vi "Circus PCs IPs.vi"(3 "error in (no error)":errorcluster, 4 "ID":string) -> (0 "error out":errorcluster, 1 "IP":string)   [LabVIEW 2026, in "TALOS.lvlib"]
doc: "This VI gives the IP of a PC, given its name, if it has been correctly inserted in the AEgIS_Config_Param.ini. If not present, it returns its ID (which is also its DNS name)."
uses:
  TALOS.lvlib
  Ancestor/Ancestor/Ancestor.lvclass/Ancestor.ctl
  Circus Root Path.vi
  TALOS Config Param.vi
  FGV/Error Memory/Get Error Description.vi
  Get PC name.vi
  Ancestor/Ancestor/Read ID.vi
  Get Class Name.vi
  <vilib>/Utility/error.llb/Clear Errors.vi
  FGV/Error Memory/Error Memory Core.vi
  <vilib>/AdvancedString/Delimited String to 1D String Array.vi
  <vilib>/AdvancedString/Delimited String to 1D String Array (string).vi
  FGV/Error Memory/Error Crt Lvl checker.vi
  FGV/Error Memory/Error Memory Core.vi/40c8088d-b597-4017-91af-faa98e00292e.vi
  FGV/Error Memory/Error Memory Core.vi/d4a3ab98-063c-4e44-b43d-fbdcfe6c2be2.vi
  Global Memory.vi
  <vilib>/Utility/LVClass/Get LV Class Name.vi
  Is in Packed Library.vi
  TALOS Root path.vi
  Read CSV worksheet.vi
  Global Constants.vi
  <vilib>/Utility/error.llb/General Error Handler.vi
  <vilib>/Utility/config.llb/Open Config Data.vi
  <vilib>/Utility/config.llb/Get Section Names.vi
  <vilib>/Utility/config.llb/Get Key Names.vi
  <vilib>/Utility/config.llb/Read Key.vi
  <vilib>/Utility/config.llb/Read Key (String).vi
  <vilib>/Utility/config.llb/Close Config Data.vi
  Ancestor/Ancestor/Ancestor.lvclass
  <vilib>/Comparison/Equal/Equal Functor/Equal Functor.lvclass
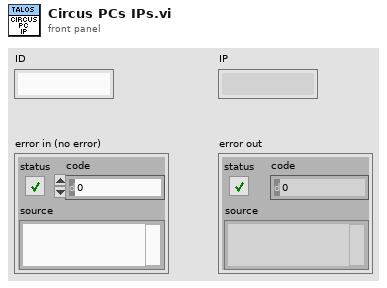
[diagram p1: front panel]
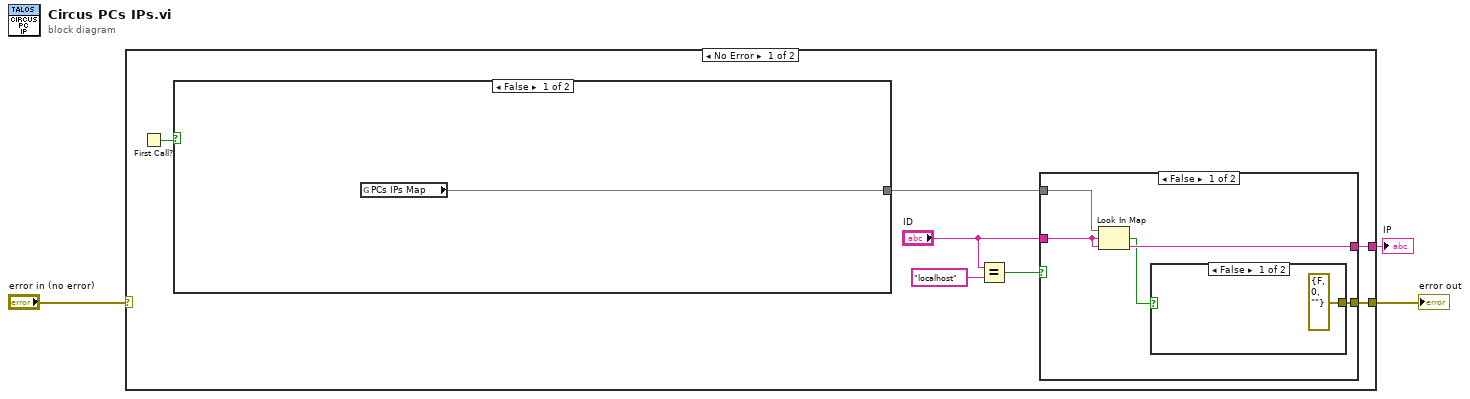
[diagram p0: block diagram]
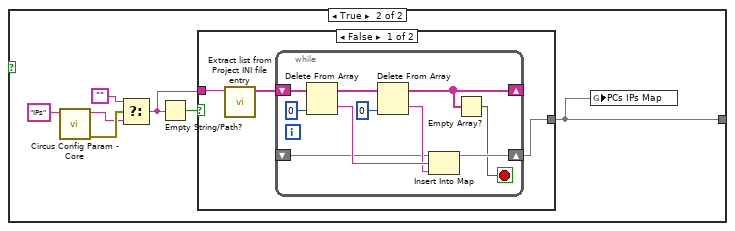
[diagram p2: hidden frame]
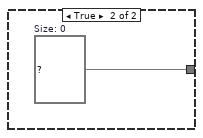
[diagram p3: hidden frame]
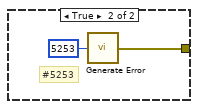
[diagram p4: hidden frame]
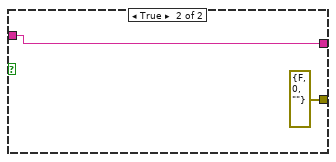
[diagram p5: hidden frame]
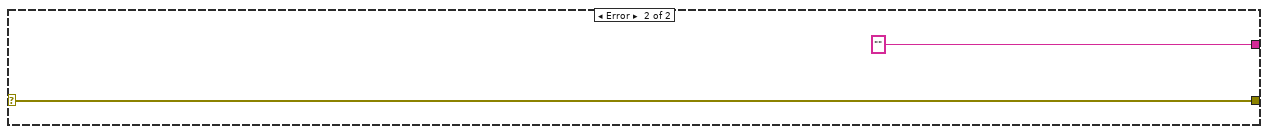
[diagram p6: hidden frame]
diagram:
  n1 = case shown="No Error" "error in (no error)" {
    selector: "error in (no error)" -> [_ w43]
    tunnel: [w8 "" ("trimmed string")] -> w3
    tunnel: [w7 w43] -> w1
    frame No Error {
      n2 = First Call?() -> (First Call?: T/F=w10:bool)
      n3 = case shown="False" w10 {
        tunnel: [w11 w12] -> w9
        frame False {
          n4 = global read "Global Memory.vi" "PCs IPs Map"() -> (w11:map{string, string})
        }
        frame True {
          n5 = call "Circus Config Param - Core.vi"("Parameter Name"="IPs") -> ("error out"=w14:errorcluster, "Output"=w13:string)  [unwired: 9 in]
          n6 = Select(t="", s=w14, f=w13) -> (s? t:f=w18:string)
          n7 = Empty String/Path?(string/path=w18) -> (empty?=w17:bool)
          n8 = case shown="False" w17 {
            tunnel: w18 -> [w20 _]
            tunnel: [w21 w32] -> w12
            frame False {
              n9 = call "Extract list from Project INI file entry.vi"("Entry from INI file"=w20) -> ("Array"=w19:string[])  [unwired: 9 in, 1 out]
              n10 = while {
                shift-right: [w25] -> w21
                shift-left: _ -> [w24]
                shift-right: [w23] -> _
                shift-left: w19 -> [w31]
                stop <- w22 stop-if-true
                n11 = Delete From Array(array=w31, index=0) -> (deleted portion=w27:string, array with subset deleted=w28:string[])  [unwired: 1 in]
                n12 = Delete From Array(array=w28, index=0) -> (deleted portion=w26:string, array with subset deleted=w23:string[])  [unwired: 1 in]
                n13 = Insert Into Map(map in=w24, key=w27, value=w26) -> (map out=w25:map{string, string})  [unwired: 2 out]
                n14 = Empty Array?(array=w23) -> (empty?=w22:bool)
              }
            }
            frame True {
              w32 = map{string, string} {}  # Size: 0
            }
          }
          n15 = global write "Global Memory.vi" "PCs IPs Map"(w12) -> ()
        }
      }
      n16 = Equal?(x="ID", y="localhost") -> (x = y?=w4:bool)
      n17 = case shown="False" w4 {
        tunnel: w9 -> [w37 _]
        tunnel: [w36 w42] -> w8
        tunnel: [w34 errorcluster {"status"=FALSE, "code"=0, "source"=""} ("error out")] -> w7
        tunnel: "ID" -> [w33 w42]
        frame False {
          n18 = Look In Map(map=w37, key=w33, default value=w33) -> (key not found?=w35:bool, value=w36:string)
          n19 = case shown="False" w35 {
            tunnel: [errorcluster {"status"=FALSE, "code"=0, "source"=""} ("error out") w40] -> w34
            frame False {
            }
            frame True {
              # "#5253"
              n20 = call "Generate Error.vi"("Error Code"=5253) -> ("error out"=w40:errorcluster)  [unwired: 6 in]
            }
          }
        }
        frame True {
        }
      }
    }
    frame Error {
    }
  }
  "IP" <- w3
  "error out" <- w1
